vi "processPacket.vi"(8 "error in (no error)":errorcluster, 10 "tcpPacket":string, 11 "tcpServerCmd in":refnum<class "TcpServerCmd.lvclass">) -> (0 "error out":errorcluster, 3 "tcpServerCmd out":refnum<class "TcpServerCmd.lvclass">)   [LabVIEW 2018, in "TcpServerCmd.lvclass"]
doc: "Process the incoming TCP packet. This could be a command or an event. If incoming packet is not command or event, just pass it to the LabVIEW Component."
uses:
  TcpServerCmd.lvclass
  home/pcortes/github/ts_labview_tcp_json/src/TcpServerBase/TcpServerBase.lvclass
  TcpServerBase/TcpServerBase.lvclass/TcpServerBase.ctl
  TcpServerBase/TcpServerBase.lvclass
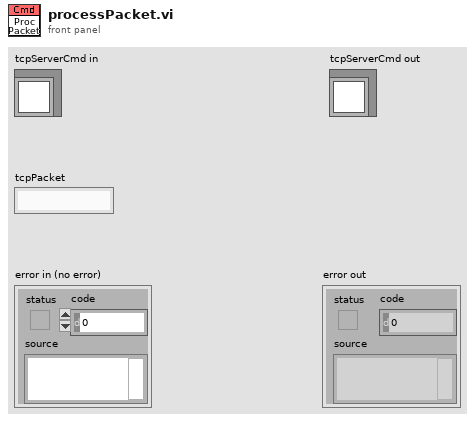
[diagram p1: front panel]
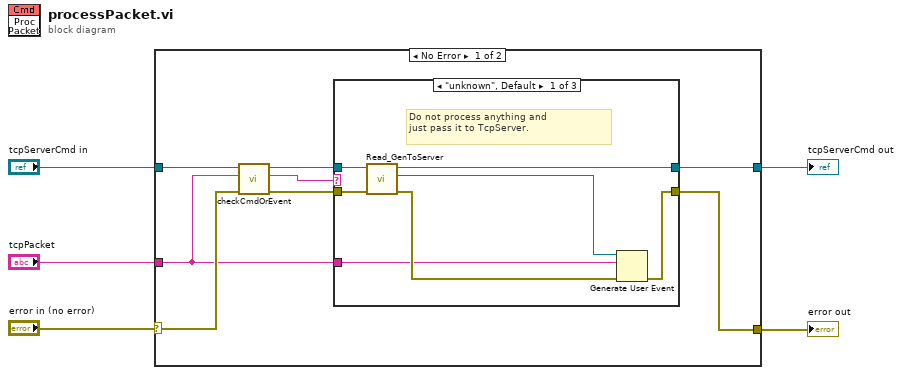
[diagram p0: block diagram]
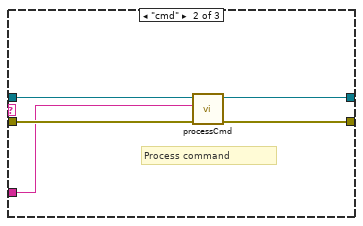
[diagram p2: hidden frame]
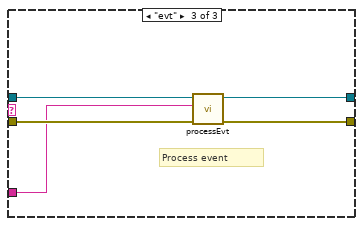
[diagram p3: hidden frame]
diagram:
  n1 = case shown="No Error" "error in (no error)" {
    selector: "error in (no error)" -> [w12 w32]
    tunnel: [w8 w32] -> w4
    tunnel: [w6 w31] -> w2
    tunnel: "tcpServerCmd in" -> [w13 w31]
    tunnel: "tcpPacket" -> [w7 _]
    frame No Error {
      n2 = call "checkCmdOrEvent.vi"("error in (no error)"=w12, "tcpPacket"=w7, "tcpServerCmd in"=w13) -> ("error out"=w10:errorcluster, "typeOfPacket"=w11:string, "tcpServerCmd out"=w9:refnum<class "TcpServerCmd.lvclass">)  [unwired: 6 in]
      n3 = case shown="\"unknown\", Default" w11 {
        tunnel: w10 -> [w17 w24 w28]
        tunnel: w9 -> [w18 w25 w30]
        tunnel: [w16 w23 w29] -> w6
        tunnel: w7 -> [w14 w22 w26]
        tunnel: [w15 w21 w27] -> w8
        frame "unknown", Default {
          # "Do not process anything and\njust pass it to TcpServer."
          n4 = call "Read_GenToServer.vi"("error in (no error)"=w17, "TcpServerBase in"=w18) -> ("error out"=w19:errorcluster, "GenToServer"=w20:refnum<user-event>, "TcpServerBase out"=w16:refnum<class "TcpServerCmd.lvclass">)  [unwired: 7 in]
          n5 = Generate User Event(user event=w20, event data cluster=w14, error in=w19) -> (error out=w15:errorcluster)  [unwired: 1 in, 1 out]
        }
        frame "cmd" {
          # "Process command"
          n6 = call "processCmd.vi"("error in (no error)"=w24, "tcpPacket"=w22, "tcpServerCmd in"=w25) -> ("error out"=w21:errorcluster, "tcpServerCmd out"=w23:refnum<class "TcpServerCmd.lvclass">)  [unwired: 7 in]
        }
        frame "evt" {
          # "Process event"
          n7 = call "processEvt.vi"("error in (no error)"=w28, "packet"=w26, "TcpServerCmd in"=w30) -> ("error out"=w27:errorcluster, "TcpServerCmd out"=w29:refnum<class "TcpServerCmd.lvclass">)  [unwired: 7 in]
        }
      }
    }
    frame Error {
    }
  }
  "error out" <- w4
  "tcpServerCmd out" <- w2
